vi "NISE.Get NVMEM Bytes.vi"(0 "SLSC Interface In":refnum<class "SLSC Interface.lvclass">, 5 "NVMEM area":refnum<k21>="$DefaultNVMEMAreas", 7 "data address":u32 format="%.0x", 9 "data size":u32, 11 "error in (no error)":errorcluster) -> (4 "SLSC Interface Out":refnum<class "SLSC Interface.lvclass">, 6 "NVMEM area out":refnum<k21>, 8 "next data address":u32 format="%.0x", 10 "data out":u8[](array[numeric]) format="%.0x", 15 "error out":errorcluster)   [LabVIEW 2016, in "SLSC Interface.lvclass"]
uses:
  SLSC Interface.lvclass
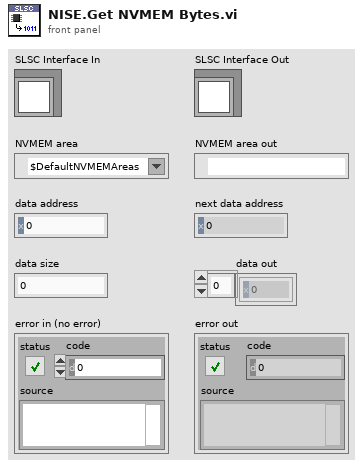
[diagram p1: front panel]
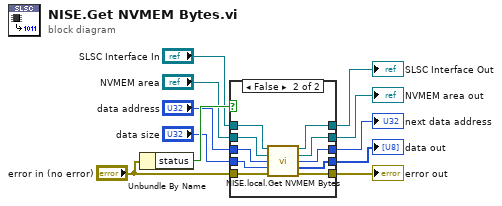
[diagram p0: block diagram]
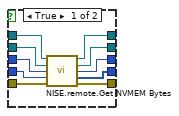
[diagram p2: hidden frame]
diagram:
  n1 = Unbundle By Name("error in (no error)") -> ("status"=w11:bool)
  n2 = case shown="False" w11 {
    tunnel: "SLSC Interface In" -> [w21 w31]
    tunnel: [w20 w30] -> w9
    tunnel: "NVMEM area" -> [w19 w29]
    tunnel: [w18 w28] -> w7
    tunnel: "data address" -> [w17 w27]
    tunnel: [w16 w26] -> w5
    tunnel: "data size" -> [w15 w25]
    tunnel: [w14 w24] -> w3
    tunnel: "error in (no error)" -> [w13 w23]
    tunnel: [w12 w22] -> w1
    frame True {
      n3 = call "NISE.remote.Get NVMEM Bytes.vi"("SLSC Remote In"=w21, "NVMEM area"=w19, "data address"=w17, "data size"=w15, "error in (no error)"=w13) -> ("SLSC Remote Out"=w20:refnum<class "SLSC Interface.lvclass">, "NVMEM area out"=w18:refnum<k21>, "next data address"=w16:u32, "data out"=w14:u8[], "error out"=w12:errorcluster)  [unwired: 6 in]
    }
    frame False {
      n4 = call "NISE.local.Get NVMEM Bytes.vi"("SLSC Local In"=w31, "NVMEM area"=w29, "data address"=w27, "data size"=w25, "error in (no error)"=w23) -> ("SLSC Local Out"=w30:refnum<class "SLSC Interface.lvclass">, "NVMEM area out"=w28:refnum<k21>, "next data address"=w26:u32, "data out"=w24:u8[], "error out"=w22:errorcluster)  [unwired: 6 in]
    }
  }
  "error out" <- w1
  "data out" <- w3
  "next data address" <- w5
  "NVMEM area out" <- w7
  "SLSC Interface Out" <- w9
